vi "WFDC CC Test Panel.vi"() -> ()   [LabVIEW 2020]
uses:
  Device Library/Cameras/IDS/IDS Controls/IDS ROI.ctl
  Hardware Configuration/Hardware Configuration Controls/Device Type.ctl
  Hardware Configuration/Hardware Configuration Controls/Device Function.ctl
  Device Library/Cameras/IDS/IDS Controls/IDS Actions.ctl
panel:
  out "Intensity Graph":dbl[][](graph)
  in  "Quit":bool
  in  "CC Half Shift":i32=20
  in  "Scan Positions":path
  in  "ROI Path":path
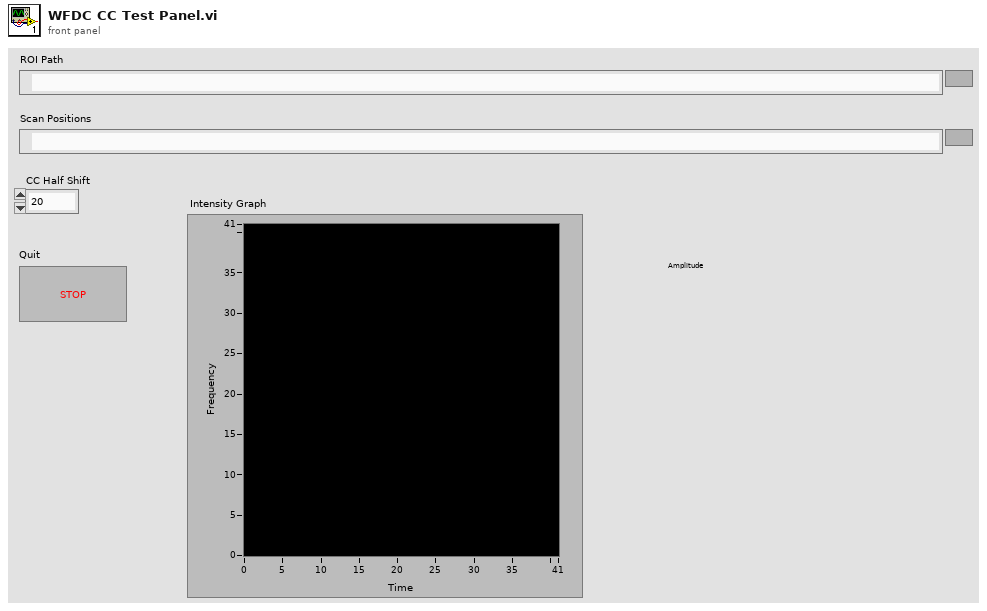
[diagram p1: front panel]
types:
  T1 = typedef "IDS Actions.ctl" = enum16{"Error Check", "Initialize", "Preview", "Record", "Abort", "Record Settings", "Set Parameter", "Get Parameter", "Set ROI", "Get ROI", "Status", "Quit"}
  T2 = typedef "Device Function.ctl" = enum16{"Primary", "Secondary", "Overview", "Wide Field Drift Correction", "642 nm Excitation", "560 nm Excitation", "940 nm Excitation", "546 nm Excitation", "488 nm Excitation", "405 nm Excitation", "Objective Drift Correction", "4Pi Objective Lock", "Objective XY", "Objective Z", "Sample XY", "Sample Coarse Z", "Sample Z", "4Pi Lower", "4Pi Upper", "Mojo", "Adj Cavity", "Line Scanning", "Alert"}
  T3 = typedef "Device Type.ctl" = enum16{"AOTF", "Camera", "Deformable Mirror", "Laser", "Microscope Base", "Shutter", "Stage", "Waveform", "FPGA", "Email", "Filter Wheel", "Spinning Disk"}
  T4 = typedef "IDS ROI.ctl" = cluster{"H Offset":i32, "V Offset":i32, "H Width":i32, "V Width":i32}
  T5 = typedef "IMAQ Image.ctl" = refnum<image>
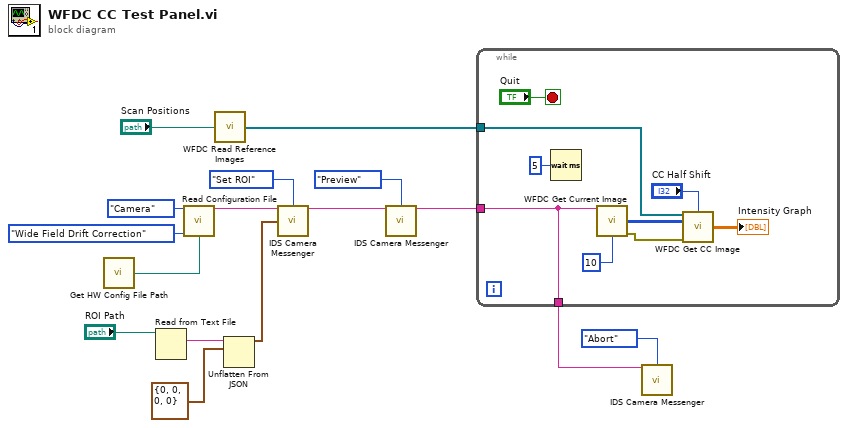
[diagram p0: block diagram]
diagram:
  n1 = call "Get HW Config File Path.vi"() -> ("File Path"=w13:path)  [unwired: 14 in, 1 out]
  n2 = Read from Text File(file (use dialog)="ROI Path") -> (text=w15:string)  [unwired: 3 in, 3 out]
  n3 = call "Read Configuration File.vi"("Device Type"=Device_Type."Camera", "Device Function"=Device_Function."Wide Field Drift Correction", "Config File Path"=w13) -> ("Unique Notifier Name"=w9:string)  [unwired: 9 in, 3 out]
  n4 = call "WFDC Read Reference Images.vi"("Scan Positions File Path"="Scan Positions") -> ("Ref Images"=w6:T5[])  [unwired: 13 in, 1 out]
  n5 = Unflatten From JSON(JSON string=w15, type and defaults=T4 {"H Offset"=0, "V Offset"=0, "H Width"=0, "V Width"=0} ("ROI Setup")) -> (value=w7:T4)  [unwired: 5 in, 1 out]
  n6 = call "IDS Camera Messenger.vi"("Notifier Name"=w9, "IDS Actions"=IDS_Actions."Set ROI", "ROI Setup"=w7) -> ("Notifier Name (Dup)"=w4:string)  [unwired: 7 in, 5 out]
  n7 = call "IDS Camera Messenger.vi"("Notifier Name"=w4, "IDS Actions"=IDS_Actions."Preview") -> ("Notifier Name (Dup)"=w3:string)  [unwired: 8 in, 5 out]
  n8 = while {
    tunnel: w3 -> [w17]
    tunnel: w6 -> [w24]
    tunnel: [w17] -> w1
    stop <- "Quit" stop-if-true
    n9 = Wait (ms)(milliseconds to wait=u32 5) -> ()  [unwired: 1 out]
    n10 = call "WFDC Get Current Image.vi"("IDS Camera Notifier Name"=w17, "Frames"=u16 10) -> ("Image - U16"=w23:u16[][], "Error"=w22:errorcluster)  [unwired: 11 in, 1 out]
    n11 = call "WFDC Get CC Image.vi"("Ref Images"=w24, "Half Shift"="CC Half Shift", "Current Image"=w23, "Error In"=w22) -> ("CC Image"=→"Intensity Graph":dbl[][])  [unwired: 10 in, 1 out]
  }
  n12 = call "IDS Camera Messenger.vi"("Notifier Name"=w1, "IDS Actions"=IDS_Actions."Abort") -> ()  [unwired: 8 in, 6 out]
